vi "Write Controller.vi"(10 "Controllers.lvlib:Abstract Controller.lvclass":refnum<class "Abstract Controller.lvclass">, 11 "User Interface in":refnum<class "User Interface.lvclass">) -> (3 "User Interface out":refnum<class "User Interface.lvclass">)   [LabVIEW 2016, in "User Interface.lvlib" / "User Interface.lvclass"]
uses:
  User Interface.lvclass
  Controllers/Abstract Controller/Abstract Controller.lvclass
  User Interface.lvclass/User Interface.ctl
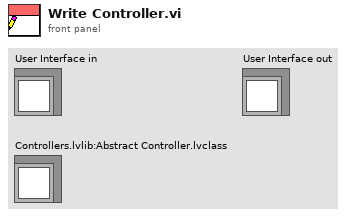
[diagram p1: front panel]
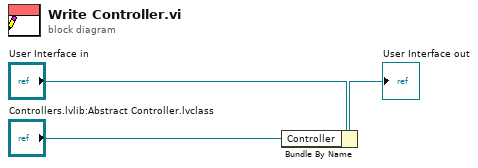
[diagram p0: block diagram]
diagram:
  n1 = Bundle By Name(cluster="User Interface in", "Controller"="Controllers.lvlib:Abstract Controller.lvclass") -> (→"User Interface out":refnum<class "User Interface.lvclass">)
